vi "Mark Target Centers.vi"(2 "Processed Image":T2(plugin-control), 3 "Target Info":T1(array[cluster])) -> (0 "Target":bool, 1 "Image Out":T2(plugin-control))   [LabVIEW 2011]
doc: "This SubVI is used to mark the target's centers in their appropriate order.\n\nThe order is left-to-right: the left target on the array on your left is Target no. 1, and the right one is 4."
panel:
  in  "Target Found?":bool
  # "These variables are used to determine whether a target is found to enable auto-search on the Robot Code."
  # "This SubVI is used to mark the target's centers in their appropriate order.\nThe order is left-to-right: the left target on the array on your left is Target no. 1, and the right one is 4."
  # "1"
  # "2"
  # "3"
  # "4"
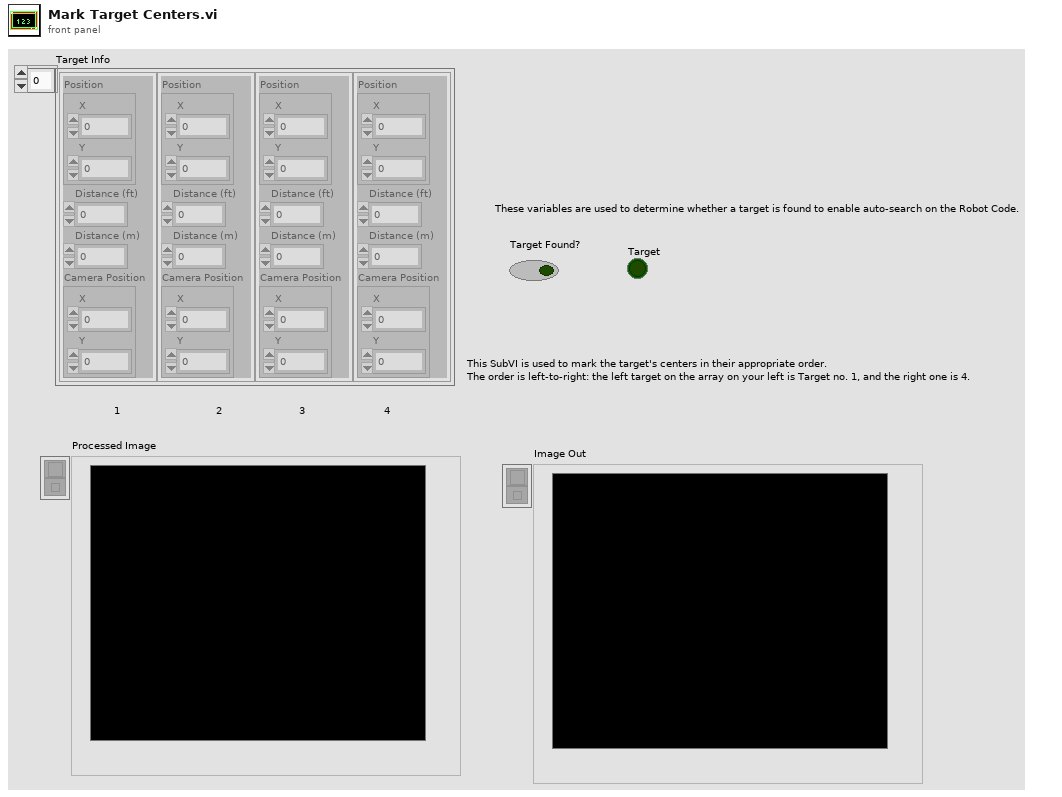
[diagram p1: front panel]
types:
  T1 = cluster{"Position":cluster{"X":dbl, "Y":dbl}, "Distance (ft)":dbl, "Distance (m)":dbl, "Camera Position":cluster{"X":dbl, "Y":dbl}}[]
  T2 = typedef "IMAQ Image.ctl" = refnum<image>
  T3 = cluster{"Position":cluster{"X":dbl, "Y":dbl}, "Distance (ft)":dbl, "Distance (m)":dbl, "Camera Position":cluster{"X":dbl, "Y":dbl}}
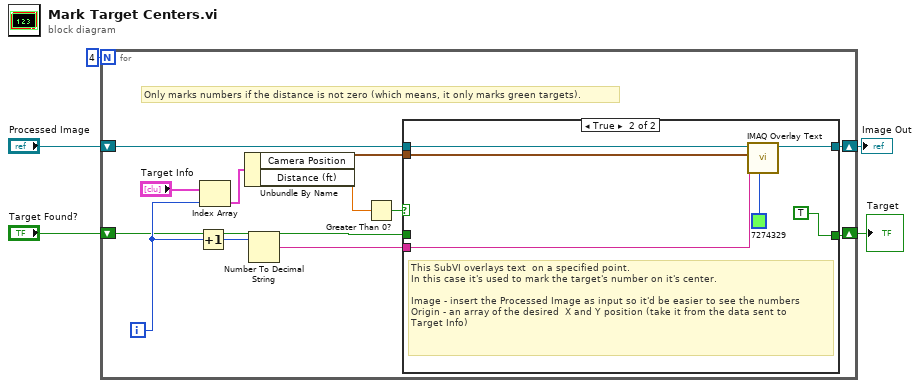
[diagram p0: block diagram]
diagram:
  n1 = for {
    N: 4 -> [_]
    shift-right: [w13] -> w3
    shift-left: "Processed Image" -> [w12]
    shift-right: [w7] -> w1
    shift-left: "Target Found?" -> [w6]
    i -> [w17]
    # "Only marks numbers if the distance is not zero (which means, it only marks green targets)."
    n2 = Increment(x=w17) -> (x+1=w16:i32)
    n3 = Index Array(array="Target Info", index=w17) -> (element=w14:T3)
    n4 = Unbundle By Name(w14) -> ("Camera Position"=w10:cluster{"X":dbl, "Y":dbl}, "Distance (ft)"=w8:dbl)
    n5 = Number To Decimal String(number=w16) -> (decimal integer string=w15:string)  [unwired: 1 in]
    n6 = Greater Than 0?(x=w8) -> (x > 0?=w9:bool)
    n7 = case shown="True" w9 {
      tunnel: w15 -> [_ w24]
      tunnel: w10 -> [_ w23]
      tunnel: [w19 w22] -> w13
      tunnel: w12 -> [w19 w21]
      tunnel: [w18 TRUE] -> w7
      tunnel: w6 -> [w18 _]
      frame False {
      }
      frame True {
        # "This SubVI overlays text  on a specified point.\nIn this case it's used to mark the target's number on it's center.\n\nImage - insert the Processed Image as input so it'd be easier to see the numbers\nOrigin - an array of the desired  X and Y position (take it from the data sent to\nTarget Info)"
        n8 = call "IMAQ Overlay Text"("Text Color (black)"=u32 7274329 ("Color"), "String"=w24, "Origin"=w23, "Image"=w21) -> ("Image Out"=w22:T2)  [unwired: 6 in, 1 out]
      }
    }
  }
  "Image Out" <- w3
  "Target" <- w1
